vi "Map_2Buttons_To_Throttle.vi"(7 "Power":dbl=1.0, 9 "Down":bool=TRUE, 10 "Up":bool=TRUE) -> (2 "Throttle":dbl)   [LabVIEW 2019]
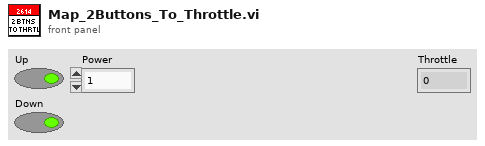
[diagram p1: front panel]
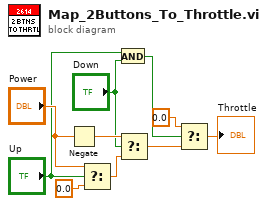
[diagram p0: block diagram]
diagram:
  n1 = Negate(x="Power") -> (-x=w7:dbl)
  n2 = Select(t="Power", s="Up", f=0.0) -> (s? t:f=w9:dbl)
  n3 = And(x="Up", y="Down") -> (x .and. y?=w6:bool)
  n4 = Select(t=w7, s="Down", f=w9) -> (s? t:f=w1:dbl)
  n5 = Select(t=0.0, s=w6, f=w1) -> (s? t:f=→"Throttle":dbl)
